vi "Main.vi"() -> ()   [LabVIEW 2019]
uses:
  controls/States.ctl
panel:
  in  "Log Results":bool
  in  "View Results":bool
  in  "Start Test":bool
  in  "Edit Configuration":bool
  in  "stop":bool
  # "User Panel"
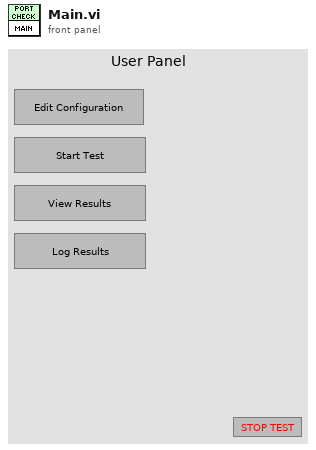
[diagram p1: front panel]
types:
  T1 = typedef "States.ctl" = enum16{"Initialize", "Stop", "Edit Configuration", "Idle", "Start Test", "View Results", "Log Results"}
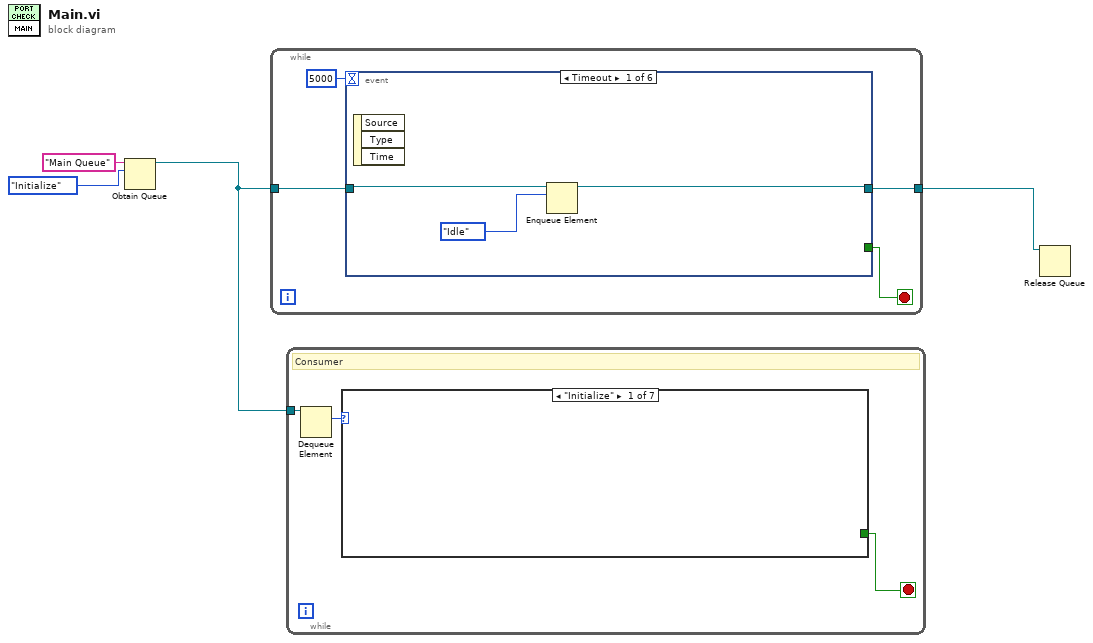
[diagram p0: block diagram]
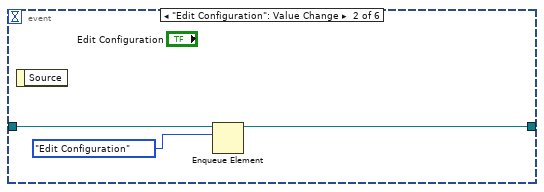
[diagram p2: hidden frame]
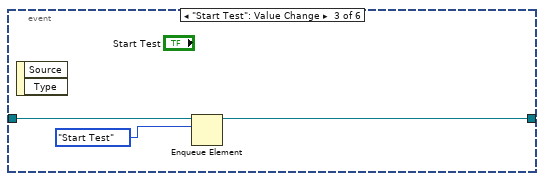
[diagram p3: hidden frame]
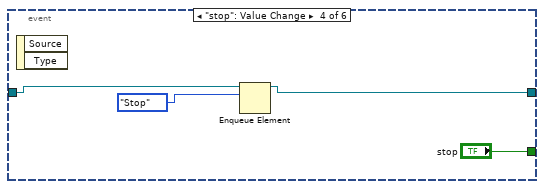
[diagram p4: hidden frame]
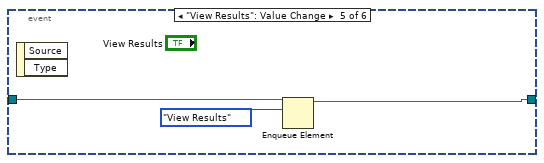
[diagram p5: hidden frame]
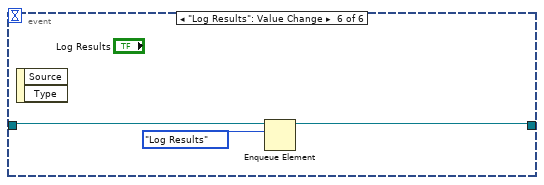
[diagram p6: hidden frame]
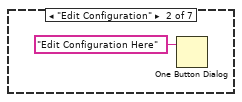
[diagram p7: hidden frame]
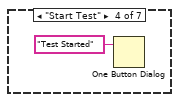
[diagram p9: hidden frame]
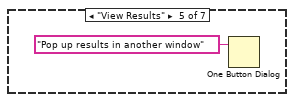
[diagram p10: hidden frame]
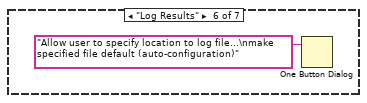
[diagram p11: hidden frame]
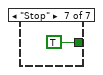
[diagram p12: hidden frame]
diagram:
  n1 = Obtain Queue(name (unnamed)="Main Queue", element data type=States."Initialize" ("States")) -> (queue out=w2:refnum<queue>)  [unwired: 3 in, 2 out]
  n2 = while {
    tunnel: w2 -> [w8]
    tunnel: [w7] -> w1
    stop <- w6 stop-if-true
    n3 = event shown="[0] Timeout" {
      selector: _ -> [_ _ _ _ _ _]
      dyn-events: _ -> [_ _ _ _ _ _]
      timeout: 5000 -> [_ _ _ _ _ _]
      tunnel: w8 -> [w11 w14 w17 w20 w23 w26]
      tunnel: [w9 w12 w15 w19 w22 w25] -> w7
      tunnel: [_ _ _ "stop" _ _] -> w6
      event Timeout {
        n4 = event-data() -> ()  [unwired: 1 in, 3 out]
        n5 = Enqueue Element(queue=w11, element=States."Idle" ("States")) -> (queue out=w9:refnum<queue>)  [unwired: 2 in, 2 out]
      }
      event "Edit Configuration": Value Change {
        n6 = event-data() -> ()  [unwired: 1 in, 1 out]
        n7 = Enqueue Element(queue=w14, element=States."Edit Configuration" ("States")) -> (queue out=w12:refnum<queue>)  [unwired: 2 in, 2 out]
      }
      event "Start Test": Value Change {
        n8 = event-data() -> ()  [unwired: 1 in, 2 out]
        n9 = Enqueue Element(queue=w17, element=States."Start Test" ("States")) -> (queue out=w15:refnum<queue>)  [unwired: 2 in, 2 out]
      }
      event "stop": Value Change {
        n10 = event-data() -> ()  [unwired: 1 in, 2 out]
        n11 = Enqueue Element(queue=w20, element=States."Stop" ("States")) -> (queue out=w19:refnum<queue>)  [unwired: 2 in, 2 out]
      }
      event "View Results": Value Change {
        n12 = event-data() -> ()  [unwired: 1 in, 2 out]
        n13 = Enqueue Element(queue=w23, element=States."View Results" ("States")) -> (queue out=w22:refnum<queue>)  [unwired: 2 in, 2 out]
      }
      event "Log Results": Value Change {
        n14 = event-data() -> ()  [unwired: 1 in, 2 out]
        n15 = Enqueue Element(queue=w26, element=States."Log Results" ("States")) -> (queue out=w25:refnum<queue>)  [unwired: 2 in, 2 out]
      }
    }
  }
  n16 = while {
    tunnel: w2 -> [w30]
    stop <- w28 stop-if-true
    # "Consumer"
    n17 = Dequeue Element(queue=w30) -> (element=w29:T1)  [unwired: 2 in, 3 out]
    n18 = case shown="\"Initialize\"" w29 {
      tunnel: [_ _ _ _ _ _ TRUE] -> w28
      frame "Initialize" {
      }
      frame "Edit Configuration" {
        n19 = One Button Dialog(message="Edit Configuration Here") -> ()  [unwired: 1 in, 1 out]
      }
      frame "Idle", Default {
      }
      frame "Start Test" {
        n20 = One Button Dialog(message="Test Started") -> ()  [unwired: 1 in, 1 out]
      }
      frame "View Results" {
        n21 = One Button Dialog(message="Pop up results in another window") -> ()  [unwired: 1 in, 1 out]
      }
      frame "Log Results" {
        n22 = One Button Dialog(message="Allow user to specify location to log file...\nmake specified file default (auto-configuration)") -> ()  [unwired: 1 in, 1 out]
      }
      frame "Stop" {
      }
    }
  }
  n23 = Release Queue(queue=w1) -> ()  [unwired: 2 in, 3 out]
